vi "create.vi"(7 "name":string, 8 "error in":errorcluster, 10 "groups":refnum<class "test-group.lvclass">[](array[class]), 11 "test-device in":refnum<class "test-device.lvclass">) -> (0 "error out":errorcluster, 3 "test-device out":refnum<class "test-device.lvclass">)   [LabVIEW 2020, in "test-device.lvclass"]
uses:
  test-device.lvclass
  test-group/test-group.lvclass
  test-device.lvclass/test-device.ctl
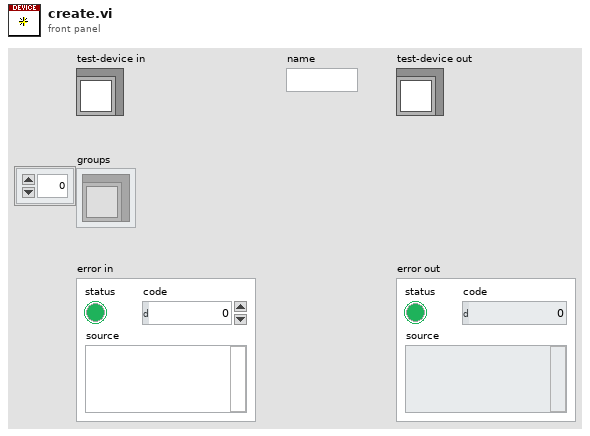
[diagram p1: front panel]
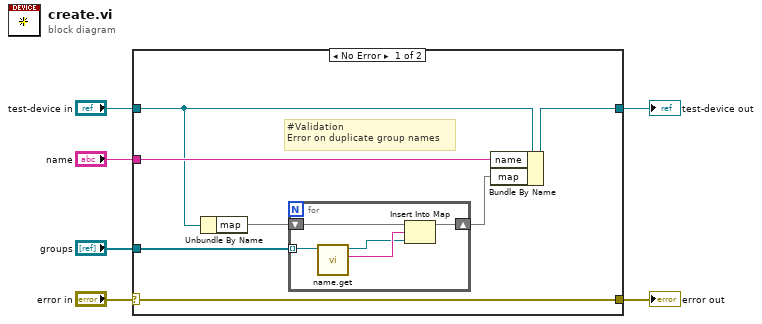
[diagram p0: block diagram]
diagram:
  n1 = case shown="No Error" "error in" {
    selector: "error in" -> [w13 w20]
    tunnel: [w13 w20] -> w5
    tunnel: [w12 w19] -> w3
    tunnel: "test-device in" -> [w9 w19]
    tunnel: "groups" -> [w11 _]
    tunnel: "name" -> [w10 _]
    frame No Error {
      # "#Validation\nError on duplicate group names"
      n2 = Unbundle By Name(w9) -> ("map"=w8:map{string, refnum<class "test-group.lvclass">})
      n3 = for {
        tunnel: w11 -> [w18] mode=indexing
        shift-right: [w15] -> w7
        shift-left: w8 -> [w14]
        n4 = call "name.get.vi"("test-group in"=w18) -> ("name"=w17:string, "test-group out"=w16:refnum<class "test-group.lvclass">)  [unwired: 9 in]
        n5 = Insert Into Map(map in=w14, key=w17, value=w16) -> (map out=w15:map{string, refnum<class "test-group.lvclass">})  [unwired: 2 out]
      }
      n6 = Bundle By Name(cluster=w9, "name"=w10, "map"=w7) -> (w12:refnum<class "test-device.lvclass">)
    }
    frame Error {
    }
  }
  "error out" <- w5
  "test-device out" <- w3
